vi "Write Device Identification.vi"(8 "error in (no error)":errorcluster, 10 "objects":cluster{"object ID":u8, "value":string}[](array[cluster]) {"object ID" format="%x"}, 11 "Modbus slave in":refnum<class "Modbus Master CR API.lvclass">) -> (0 "error out":errorcluster, 3 "Modbus slave out":refnum<class "Modbus Master CR API.lvclass">)   [LabVIEW 2021, in "Modbus Master CR API.lvclass"]
doc: "Writes the device identification of a Modbus slave. Device identification consists of data elements called objects. Each object has an identification number and stores Modbus slave information."
uses:
  Modbus Master CR API.lvclass
  Modbus Master CR API.lvclass/Modbus Master CR API.ctl
  Data Model/Device Data Model.lvclass
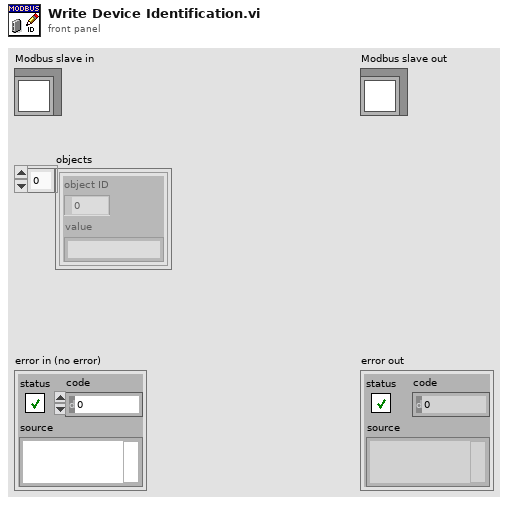
[diagram p1: front panel]
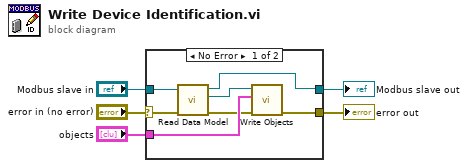
[diagram p0: block diagram]
diagram:
  n1 = case shown="No Error" "error in (no error)" {
    selector: "error in (no error)" -> [w10 w14]
    tunnel: [w6 w13] -> w5
    tunnel: "Modbus slave in" -> [w7 w13]
    tunnel: [w12 w14] -> w3
    tunnel: "objects" -> [w11 _]
    frame No Error {
      n2 = call "Read Data Model.vi"("error in (no error)"=w10, "Modbus slave in"=w7) -> ("error out"=w9:errorcluster, "device data model"=w8:refnum<class "Device Data Model.lvclass">, "Modbus slave out"=w6:refnum<class "Modbus Master CR API.lvclass">)  [unwired: 7 in]
      n3 = call-dynamic "Write Objects.vi"("error in"=w9, "Objects"=w11, "device data model in"=w8) -> ("error out"=w12:errorcluster)  [unwired: 7 in, 1 out]
    }
    frame Error {
    }
  }
  "error out" <- w3
  "Modbus slave out" <- w5
